vi "ConvertStrTimeToSecond.vi"(11 "string time":string) -> (3 "second":dbl)   [LabVIEW 2018, in "Library-DataConvert.lvlib"]
uses:
  Library-DataConvert.lvlib
panel:
  out "에러 출력":errorcluster
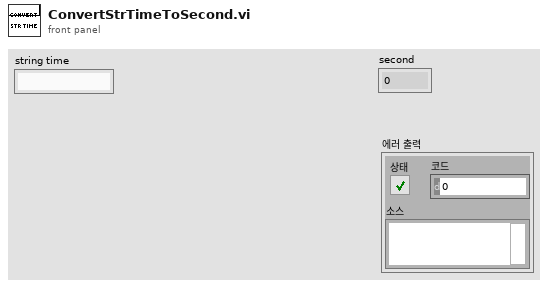
[diagram p1: front panel]
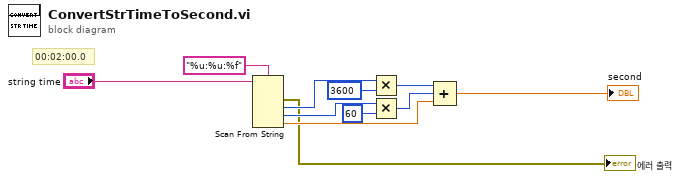
[diagram p0: block diagram]
diagram:
  # "00:02:00.0"
  n1 = Scan From String(format string="%u:%u:%f" ("포맷 문자열"), input string="string time") -> (error out=→"에러 출력":errorcluster, output 1=w4:u32, output 2=w9:u32, output 3=w6:dbl)  [unwired: 5 in, 2 out]
  n2 = Multiply(x=w4, y=u32 3600) -> (x*y=w8:u32)
  n3 = Multiply(x=w9, y=u32 60) -> (x*y=w7:u32)
  n4 = Compound Arithmetic op=ADD(w8, w7, w6) -> (→"second":dbl)
